vi "ConfigPanel.vi"(8 "ErrorIn":errorcluster, 11 "ClusterIn":T4={"Admin"={"Lvl"=enum."Admin", "Pwd"=""}, "RTConfig"={"Arm"=FALSE, "Number"=0.0, "String"=""}, "SMS"={"Enbl?"=FALSE, "Addr"=[]}, "FPGA"={"Target"=enum."4", "Channel"=enum."4", "Ref1"=refnum, "Ref2"=refnum}, "Config"={"UsrCfg"={"Paths"={"CfgFile"=path "", "LogFolder"=path "", "LogFile"=path "", "NAS path"=path "", "ThreshFile"=path "", "RedunFolder"=path ""}, "SampleRate"=12500.0}, "FP_User"={"#NoiseSums"=1, "Max_df"=1, "AvgAvg"=FALSE, "#Avg"=1, "AutoCenter"=FALSE, "Inclin"={"Vmin"=0.0, "Vmax"=0.0, "Angle_min"=0.0, "Angle_max"=0.0, "Offset"=0.0, "Pos_Neg"=FALSE}, "1"={"Cal_"={"Fine"=0.999969482421875, "Coarse_"=10000.0}, "Beac"={"Fine"=4194303.0, "Coarse_"=1.0}, "Scale"={"Step4"=10000.0, "Step5"=4194303.0, "Step6"=1.0, "Step7"=10000.0}, "Offset"=1.0, "Scale_Noise"=12500.0, "Scale_Step1"=65535.0, "Scale_In_RT"=1.0, "ScaleMeas"=0.999969482421875, "FreqsToRemove"=[0, 1633], "Width"=[0, 1633], "ScaleMeasEnum"=enum."50", "FilterEnab"=enum."Step 1"}, "2"={"Cal_"={"Fine"=0.000213623046875, "Coarse_"=4194303.0}, "Beac"={"Fine"=0.000213623046875, "Coarse_"=4194303.0}, "Scale"={"Step4"=0.0, "Step5"=4194303.0, "Step6"=1.0, "Step7"=10000.0}, "Offset"=0.0, "Scale_Noise"=4194303.0, "Scale_Step1"=65535.0, "Scale_In_RT"=1.0, "ScaleMeas"=0.999969482421875, "FreqsToRemove"=[0, 1633], "Width"=[0, 1633], "ScaleMeasEnum"=enum."50", "FilterEnab"=enum."Step 1"}, "3"={"Cal_"={"Fine"=0.000213623046875, "Coarse_"=4194303.0}, "Beac"={"Fine"=0.000213623046875, "Coarse_"=4194303.0}, "Scale"={"Step4"=0.0, "Step5"=4194303.0, "Step6"=1.0, "Step7"=10000.0}, "Offset"=0.0, "Scale_Noise"=4194303.0, "Scale_Step1"=65535.0, "Scale_In_RT"=1.0, "ScaleMeas"=0.999969482421875, "FreqsToRemove"=[0, 1633], "Width"=[0, 1633], "ScaleMeasEnum"=enum."50", "FilterEnab"=enum."Step 1"}, "4"={"Cal_"={"Fine"=0.000213623046875, "Coarse_"=4194303.0}, "Beac"={"Fine"=0.000213623046875, "Coarse_"=4194303.0}, "Scale"={"Step4"=0.0, "Step5"=4194303.0, "Step6"=1.0, "Step7"=10000.0}, "Offset"=0.0, "Scale_Noise"=4194303.0, "Scale_Step1"=1.0, "Scale_In_RT"=10000.0, "ScaleMeas"=0.999969482421875, "FreqsToRemove"=[0, 1633], "Width"=[0, 1633], "ScaleMeasEnum"=enum."50", "FilterEnab"=enum."Step 1"}, "Target to Probe"=enum."4", "SNR_Thresh"=1.0, "Paths"={"CfgFile"=path "", "LogFolder"=path "", "LogFile"=path "", "NAS path"=path "", "ThreshFile"=path "", "RedunFolder"=path ""}, "Connex_Location"="", "SimulateFPGA"=FALSE, "Deadband"=0.0}}, "Stat"={"SysState"=enum."Init", "TrackRate"=FALSE, "AutoCentr"=FALSE}, "Alarm"={"TC13"={"Enbl"=FALSE, "ErrsAndWarns"={0.0, 5.663716814159292, 7.168141592920354, 8.584070796460177}}, "AI1"={"Enbl"=FALSE, "ErrsAndWarns"={0.0, 5.663716814159292, 7.168141592920354, 8.584070796460177}}, "AI2"={"Enbl"=FALSE, "ErrsAndWarns"={0.0, 5.663716814159292, 7.168141592920354, 8.584070796460177}}, "AI3"={"Enbl"=FALSE, "ErrsAndWarns"={0.0, 5.663716814159292, 7.168141592920354, 8.584070796460177}}, "AI4"={"Enbl"=FALSE, "ErrsAndWarns"={0.0, 5.663716814159292, 7.168141592920354, 8.584070796460177}}, "AI5"={"Enbl"=FALSE, "ErrsAndWarns"={0.0, 5.663716814159292, 7.168141592920354, 8.584070796460177}}, "AI6"={"Enbl"=FALSE, "ErrsAndWarns"={0.0, 5.663716814159292, 7.168141592920354, 8.584070796460177}}, "AI18"={"Enbl"=FALSE, "ErrsAndWarns"={0.0, 5.663716814159292, 7.168141592920354, 8.584070796460177}}, "AI19"={"Enbl"=FALSE, "ErrsAndWarns"={0.0, 5.663716814159292, 7.168141592920354, 8.584070796460177}}, "TE1"={"Enbl"=FALSE, "ErrsAndWarns"={0.0, 5.663716814159292, 7.168141592920354, 8.584070796460177}}, "TE2"={"Enbl"=TRUE, "ErrsAndWarns"={0.0, 5.663716814159292, 7.168141592920354, 8.584070796460177}}, "TE3"={"Enbl"=FALSE, "ErrsAndWarns"={0.0, 5.663716814159292, 7.168141592920354, 8.584070796460177}}, "ADAM1"={"Enbl"=FALSE, "ErrsAndWarns"={0.0, 5.663716814159292, 7.168141592920354, 8.584070796460177}}, "ADAM2"={"Enbl"=FALSE, "ErrsAndWarns"={0.0, 5.663716814159292, 7.168141592920354, 8.584070796460177}}, "ADAM3"={"Enbl"=FALSE, "ErrsAndWarns"={0.0, 5.663716814159292, 7.168141592920354, 8.584070796460177}}, "ADAM4"={"Enbl"=FALSE, "ErrsAndWarns"={0.0, 5.663716814159292, 7.168141592920354, 8.584070796460177}}, "72CoBeacFreq"={"Enbl"=FALSE, "ErrsAndWarns"={0.0, 5.663716814159292, 7.168141592920354, 8.584070796460177}}, "72CoCalFreq"={"Enbl"=FALSE, "ErrsAndWarns"={0.0, 5.663716814159292, 7.168141592920354, 8.584070796460177}}, "84CoBeacFreq"={"Enbl"=FALSE, "ErrsAndWarns"={0.0, 5.663716814159292, 7.168141592920354, 8.584070796460177}}, "84CoCalFreq"={"Enbl"=FALSE, "ErrsAndWarns"={0.0, 5.663716814159292, 7.168141592920354, 8.584070796460177}}, "72Co_CalTonePwr"={"Enbl"=FALSE, "ErrsAndWarns"={0.0, 5.663716814159292, 7.168141592920354, 8.584070796460177}}, "72X_CalTonePwr"={"Enbl"=FALSE, "ErrsAndWarns"={0.0, 5.663716814159292, 7.168141592920354, 8.584070796460177}}, "84Co_CalTonePwr"={"Enbl"=FALSE, "ErrsAndWarns"={0.0, 5.663716814159292, 7.168141592920354, 8.584070796460177}}, "84X_CalTonePwr"={"Enbl"=FALSE, "ErrsAndWarns"={0.0, 5.663716814159292, 7.168141592920354, 8.584070796460177}}}} {"Alarm"."84X_CalTonePwr"."ErrsAndWarns" scale=-120.0..-45.0; "Alarm"."72X_CalTonePwr"."ErrsAndWarns" scale=-120.0..-45.0; "Alarm"."84Co_CalTonePwr"."ErrsAndWarns" scale=-120.0..-45.0; "Alarm"."72Co_CalTonePwr"."ErrsAndWarns" scale=-120.0..-45.0; "Alarm"."84CoCalFreq"."ErrsAndWarns" scale=24.9..25.1; "Alarm"."84CoBeacFreq"."ErrsAndWarns" scale=25.5..27.0; "Alarm"."72CoCalFreq"."ErrsAndWarns" scale=24.9..25.1; "Alarm"."72CoBeacFreq"."ErrsAndWarns" scale=25.5..27.0; "Alarm"."ADAM4"."ErrsAndWarns" scale=30.0..52.0; "Alarm"."ADAM3"."ErrsAndWarns" scale=30.0..52.0; "Alarm"."ADAM2"."ErrsAndWarns" scale=30.0..52.0; "Alarm"."ADAM1"."ErrsAndWarns" scale=30.0..52.0; "Alarm"."TE3"."ErrsAndWarns" scale=30.0..52.0; "Alarm"."TE2"."ErrsAndWarns" scale=30.0..52.0; "Alarm"."TE1"."ErrsAndWarns" scale=20.0..52.0; "Alarm"."AI19"."ErrsAndWarns" scale=0.0..60.0; "Alarm"."AI18"."ErrsAndWarns" scale=-10.0..10.0; "Alarm"."AI6"."ErrsAndWarns" scale=0.0..35.0; "Alarm"."AI5"."ErrsAndWarns" scale=0.0..20.0; "Alarm"."AI4"."ErrsAndWarns" scale=0.0..15.0; "Alarm"."AI3"."ErrsAndWarns" scale=0.0..10.0; "Alarm"."AI2"."ErrsAndWarns" scale=0.0..10.0; "Alarm"."TC13"."ErrsAndWarns" scale=-10.0..40.0; "Config"."FP_User"."Deadband" format="%#.0f"}) -> (0 "ErrorOut":errorcluster, 3 "ClusterOut":T4={"Admin"={"Lvl"=enum."Admin", "Pwd"=""}, "RTConfig"={"Arm"=FALSE, "Number"=0.0, "String"=""}, "SMS"={"Enbl?"=FALSE, "Addr"=[]}, "FPGA"={"Target"=enum."4", "Channel"=enum."4", "Ref1"=refnum, "Ref2"=refnum}, "Config"={"UsrCfg"={"Paths"={"CfgFile"=path "", "LogFolder"=path "", "LogFile"=path "", "NAS path"=path "", "ThreshFile"=path "", "RedunFolder"=path ""}, "SampleRate"=12500.0}, "FP_User"={"#NoiseSums"=1, "Max_df"=1, "AvgAvg"=FALSE, "#Avg"=1, "AutoCenter"=FALSE, "Inclin"={"Vmin"=0.0, "Vmax"=0.0, "Angle_min"=0.0, "Angle_max"=0.0, "Offset"=0.0, "Pos_Neg"=FALSE}, "1"={"Cal_"={"Fine"=0.999969482421875, "Coarse_"=10000.0}, "Beac"={"Fine"=4194303.0, "Coarse_"=1.0}, "Scale"={"Step4"=10000.0, "Step5"=4194303.0, "Step6"=1.0, "Step7"=10000.0}, "Offset"=1.0, "Scale_Noise"=12500.0, "Scale_Step1"=65535.0, "Scale_In_RT"=1.0, "ScaleMeas"=0.999969482421875, "FreqsToRemove"=[0, 1633], "Width"=[0, 1633], "ScaleMeasEnum"=enum."50", "FilterEnab"=enum."Step 1"}, "2"={"Cal_"={"Fine"=0.000213623046875, "Coarse_"=4194303.0}, "Beac"={"Fine"=0.000213623046875, "Coarse_"=4194303.0}, "Scale"={"Step4"=0.0, "Step5"=4194303.0, "Step6"=1.0, "Step7"=10000.0}, "Offset"=0.0, "Scale_Noise"=4194303.0, "Scale_Step1"=65535.0, "Scale_In_RT"=1.0, "ScaleMeas"=0.999969482421875, "FreqsToRemove"=[0, 1633], "Width"=[0, 1633], "ScaleMeasEnum"=enum."50", "FilterEnab"=enum."Step 1"}, "3"={"Cal_"={"Fine"=0.000213623046875, "Coarse_"=4194303.0}, "Beac"={"Fine"=0.000213623046875, "Coarse_"=4194303.0}, "Scale"={"Step4"=0.0, "Step5"=4194303.0, "Step6"=1.0, "Step7"=10000.0}, "Offset"=0.0, "Scale_Noise"=4194303.0, "Scale_Step1"=65535.0, "Scale_In_RT"=1.0, "ScaleMeas"=0.999969482421875, "FreqsToRemove"=[0, 1633], "Width"=[0, 1633], "ScaleMeasEnum"=enum."50", "FilterEnab"=enum."Step 1"}, "4"={"Cal_"={"Fine"=0.000213623046875, "Coarse_"=4194303.0}, "Beac"={"Fine"=0.000213623046875, "Coarse_"=4194303.0}, "Scale"={"Step4"=0.0, "Step5"=4194303.0, "Step6"=1.0, "Step7"=10000.0}, "Offset"=0.0, "Scale_Noise"=4194303.0, "Scale_Step1"=1.0, "Scale_In_RT"=10000.0, "ScaleMeas"=0.999969482421875, "FreqsToRemove"=[0, 1633], "Width"=[0, 1633], "ScaleMeasEnum"=enum."50", "FilterEnab"=enum."Step 1"}, "Target to Probe"=enum."4", "SNR_Thresh"=1.0, "Paths"={"CfgFile"=path "", "LogFolder"=path "", "LogFile"=path "", "NAS path"=path "", "ThreshFile"=path "", "RedunFolder"=path ""}, "Connex_Location"="", "SimulateFPGA"=FALSE, "Deadband"=0.0}}, "Stat"={"SysState"=enum."Init", "TrackRate"=FALSE, "AutoCentr"=FALSE}, "Alarm"={"TC13"={"Enbl"=FALSE, "ErrsAndWarns"={0.0, 5.663716814159292, 7.168141592920354, 8.584070796460177}}, "AI1"={"Enbl"=FALSE, "ErrsAndWarns"={0.0, 5.663716814159292, 7.168141592920354, 8.584070796460177}}, "AI2"={"Enbl"=FALSE, "ErrsAndWarns"={0.0, 5.663716814159292, 7.168141592920354, 8.584070796460177}}, "AI3"={"Enbl"=FALSE, "ErrsAndWarns"={0.0, 5.663716814159292, 7.168141592920354, 8.584070796460177}}, "AI4"={"Enbl"=FALSE, "ErrsAndWarns"={0.0, 5.663716814159292, 7.168141592920354, 8.584070796460177}}, "AI5"={"Enbl"=FALSE, "ErrsAndWarns"={0.0, 5.663716814159292, 7.168141592920354, 8.584070796460177}}, "AI6"={"Enbl"=FALSE, "ErrsAndWarns"={0.0, 5.663716814159292, 7.168141592920354, 8.584070796460177}}, "AI18"={"Enbl"=FALSE, "ErrsAndWarns"={0.0, 5.663716814159292, 7.168141592920354, 8.584070796460177}}, "AI19"={"Enbl"=FALSE, "ErrsAndWarns"={0.0, 5.663716814159292, 7.168141592920354, 8.584070796460177}}, "TE1"={"Enbl"=FALSE, "ErrsAndWarns"={0.0, 5.663716814159292, 7.168141592920354, 8.584070796460177}}, "TE2"={"Enbl"=TRUE, "ErrsAndWarns"={0.0, 5.663716814159292, 7.168141592920354, 8.584070796460177}}, "TE3"={"Enbl"=FALSE, "ErrsAndWarns"={0.0, 5.663716814159292, 7.168141592920354, 8.584070796460177}}, "ADAM1"={"Enbl"=FALSE, "ErrsAndWarns"={0.0, 5.663716814159292, 7.168141592920354, 8.584070796460177}}, "ADAM2"={"Enbl"=FALSE, "ErrsAndWarns"={0.0, 5.663716814159292, 7.168141592920354, 8.584070796460177}}, "ADAM3"={"Enbl"=FALSE, "ErrsAndWarns"={0.0, 5.663716814159292, 7.168141592920354, 8.584070796460177}}, "ADAM4"={"Enbl"=FALSE, "ErrsAndWarns"={0.0, 5.663716814159292, 7.168141592920354, 8.584070796460177}}, "72CoBeacFreq"={"Enbl"=FALSE, "ErrsAndWarns"={0.0, 5.663716814159292, 7.168141592920354, 8.584070796460177}}, "72CoCalFreq"={"Enbl"=FALSE, "ErrsAndWarns"={0.0, 5.663716814159292, 7.168141592920354, 8.584070796460177}}, "84CoBeacFreq"={"Enbl"=FALSE, "ErrsAndWarns"={0.0, 5.663716814159292, 7.168141592920354, 8.584070796460177}}, "84CoCalFreq"={"Enbl"=FALSE, "ErrsAndWarns"={0.0, 5.663716814159292, 7.168141592920354, 8.584070796460177}}, "72Co_CalTonePwr"={"Enbl"=FALSE, "ErrsAndWarns"={0.0, 5.663716814159292, 7.168141592920354, 8.584070796460177}}, "72X_CalTonePwr"={"Enbl"=FALSE, "ErrsAndWarns"={0.0, 5.663716814159292, 7.168141592920354, 8.584070796460177}}, "84Co_CalTonePwr"={"Enbl"=FALSE, "ErrsAndWarns"={0.0, 5.663716814159292, 7.168141592920354, 8.584070796460177}}, "84X_CalTonePwr"={"Enbl"=FALSE, "ErrsAndWarns"={0.0, 5.663716814159292, 7.168141592920354, 8.584070796460177}}}} {"Alarm"."84X_CalTonePwr"."ErrsAndWarns" scale=-120.0..-45.0; "Alarm"."72X_CalTonePwr"."ErrsAndWarns" scale=-120.0..-45.0; "Alarm"."84Co_CalTonePwr"."ErrsAndWarns" scale=-120.0..-45.0; "Alarm"."72Co_CalTonePwr"."ErrsAndWarns" scale=-120.0..-45.0; "Alarm"."84CoCalFreq"."ErrsAndWarns" scale=24.9..25.1; "Alarm"."84CoBeacFreq"."ErrsAndWarns" scale=25.5..27.0; "Alarm"."72CoCalFreq"."ErrsAndWarns" scale=24.9..25.1; "Alarm"."72CoBeacFreq"."ErrsAndWarns" scale=25.5..27.0; "Alarm"."ADAM4"."ErrsAndWarns" scale=30.0..52.0; "Alarm"."ADAM3"."ErrsAndWarns" scale=30.0..52.0; "Alarm"."ADAM2"."ErrsAndWarns" scale=30.0..52.0; "Alarm"."ADAM1"."ErrsAndWarns" scale=30.0..52.0; "Alarm"."TE3"."ErrsAndWarns" scale=30.0..52.0; "Alarm"."TE2"."ErrsAndWarns" scale=30.0..52.0; "Alarm"."TE1"."ErrsAndWarns" scale=20.0..52.0; "Alarm"."AI19"."ErrsAndWarns" scale=0.0..60.0; "Alarm"."AI18"."ErrsAndWarns" scale=-10.0..10.0; "Alarm"."AI6"."ErrsAndWarns" scale=0.0..35.0; "Alarm"."AI5"."ErrsAndWarns" scale=0.0..20.0; "Alarm"."AI4"."ErrsAndWarns" scale=0.0..15.0; "Alarm"."AI3"."ErrsAndWarns" scale=0.0..10.0; "Alarm"."AI2"."ErrsAndWarns" scale=0.0..10.0; "Alarm"."TC13"."ErrsAndWarns" scale=-10.0..40.0; "Config"."FP_User"."Deadband" format="%#.0f"})   [LabVIEW 2018]
doc: "This modal dialog allows the user to enter configuration data that is saved from one run to the next. This is useful for maintaining information such as instrument settings, display preferences, etc.\n\nIn general, each control on this panel should be Type-Def'd and saved to an INI file whenever the user clicks the OK button.\n\nCopyright © 2019 Epimedia, Inc. All Rights Reserved.\n\nThe Epimedia Application Library is Copyright © 2009-2019 Epimedia, Inc. \nAll Rights Reserved. Used under license."
uses:
  Controls/MasterCluster.ctl
  Controls/Clusts/AdminCluster.ctl
  Controls/UserLevelEnum.ctl
  Controls/RT_Config.ctl
  Controls/SMSDataCluster.ctl
  Controls/Clusts/FPGA_Config_Clust.ctl
  Controls/Enums/TargetNumber.ctl
  Controls/Clusts/Config_Clust.ctl
  Controls/Clusts/UserConfig.ctl
  Controls/PathsCluster.ctl
  Controls/Clusts/FrontPanel_UserConfig.ctl
  Controls/Clusts/Inclinometer_User_Cfg.ctl
  Controls/Clusts/FP_UserTargetConfig.ctl
  Controls/Clusts/FreqShift.ctl
  Controls/Clusts/FPGA_Scale.ctl
  Controls/Enums/ScaleMeasure.ctl
  Controls/RadioButtons/FilterEnableRadio.ctl
  Controls/SystemStatusCluster.ctl
  Controls/SystemStateEnum.ctl
  Controls/Clusts/AlarmSettingsClust.ctl
  Controls/Clusts/AlarmThresh_OneChan.ctl
  Queue/ConfigQueueElements.ctl
panel:
  in  "Paths":T1
  in  "User":T2
  in  "Cancel":bool
  in  "OK":bool
  # "Copyright © 2019 Epimedia, Inc. All Rights Reserved.\n\nThe Epimedia Application Library is Copyright © 2009-2019 Epimedia, Inc. \nAll Rights Reserved. Used under license."
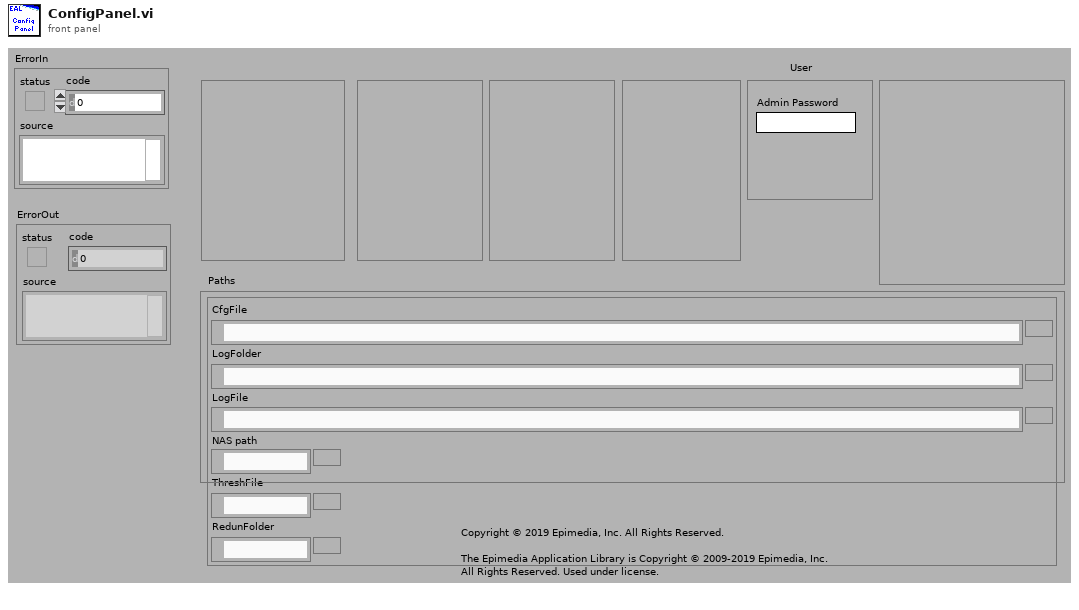
[diagram p1: front panel]
types:
  T1 = typedef "PathsCluster.ctl" = cluster{"CfgFile":path, "LogFolder":path, "LogFile":path, "NAS path":path, "ThreshFile":path, "RedunFolder":path}
  T2 = typedef "AdminCluster.ctl" = cluster{"Lvl":T3, "Pwd":string}
  T3 = typedef "UserLevelEnum.ctl" = enum16{"Admin", "Operator"}
  T4 = typedef "MasterCluster.ctl" = cluster{"Admin":T2, "RTConfig":T5, "SMS":T6, "FPGA":T7, "Config":T9, "Stat":T18, "Alarm":T20}
  T5 = typedef "RT_Config.ctl" = cluster{"Arm":bool, "Number":dbl, "String":string}
  T6 = typedef "SMSDataCluster.ctl" = cluster{"Enbl?":bool, "Addr":string[]}
  T7 = typedef "FPGA_Config_Clust.ctl" = cluster{"Target":T8, "Channel":T8, "Ref1":refnum<k20>, "Ref2":refnum<k20>}
  T8 = typedef "TargetNumber.ctl" = enum16{"1", "2", "3", "4"}
  T9 = typedef "Config_Clust.ctl" = cluster{"UsrCfg":T10, "FP_User":T11}
  T10 = typedef "UserConfig.ctl" = cluster{"Paths":T1, "SampleRate":dbl}
  T11 = typedef "FrontPanel_UserConfig.ctl" = cluster{"#NoiseSums":u32, "Max_df":u32, "AvgAvg":bool, "#Avg":u16, "AutoCenter":bool, "Inclin":T12, "1":T13, "2":T13, "3":T13, "4":T13, "Target to Probe":T8, "SNR_Thresh":dbl, "Paths":T1, "Connex_Location":string, "SimulateFPGA":bool, "Deadband":dbl}
  T12 = typedef "Inclinometer_User_Cfg.ctl" = cluster{"Vmin":dbl, "Vmax":dbl, "Angle_min":dbl, "Angle_max":dbl, "Offset":dbl, "Pos_Neg":bool}
  T13 = typedef "FP_UserTargetConfig.ctl" = cluster{"Cal_":T14, "Beac":T14, "Scale":T15, "Offset":fxp<+/-,16,16>, "Scale_Noise":fxp<+/-,30,30>, "Scale_Step1":fxp<+/-,17,17>, "Scale_In_RT":ext, "ScaleMeas":fxp<+/-,16,1>, "FreqsToRemove":i32[], "Width":i32[], "ScaleMeasEnum":T16, "FilterEnab":T17}
  T14 = typedef "FreqShift.ctl" = cluster{"Fine":dbl, "Coarse_":dbl}
  T15 = typedef "FPGA_Scale.ctl" = cluster{"Step4":fxp<+/-,23,23>, "Step5":fxp<+/-,23,23>, "Step6":fxp<+/-,23,23>, "Step7":fxp<+/-,23,23>}
  T16 = typedef "ScaleMeasure.ctl" = enum16{"1", "10", "50", "42"}
  T17 = typedef "FilterEnableRadio.ctl" = enum32{"None", "Step 1", "Frequency Shift", "Step 4", "Step 5", "Step 6", "Step 7"}
  T18 = typedef "SystemStatusCluster.ctl" = cluster{"SysState":T19, "TrackRate":bool, "AutoCentr":bool}
  T19 = typedef "SystemStateEnum.ctl" = enum16{"Init", "Idle", "Running", "System Fault", "System Error", "Exit"}
  T20 = typedef "AlarmSettingsClust.ctl" = cluster{"TC13":T21, "AI1":T21, "AI2":T21, "AI3":T21, "AI4":T21, "AI5":T21, "AI6":T21, "AI18":T21, "AI19":T21, "TE1":T21, "TE2":T21, "TE3":T21, "ADAM1":T21, "ADAM2":T21, "ADAM3":T21, "ADAM4":T21, "72CoBeacFreq":T21, "72CoCalFreq":T21, "84CoBeacFreq":T21, "84CoCalFreq":T21, "72Co_CalTonePwr":T21, "72X_CalTonePwr":T21, "84Co_CalTonePwr":T21, "84X_CalTonePwr":T21}
  T21 = typedef "AlarmThresh_OneChan.ctl" = cluster{"Enbl":bool, "ErrsAndWarns":cluster{dbl, dbl, dbl, dbl}}
  T22 = typedef "ConfigQueueElements.ctl" = enum16{"Initialize", "OK", "Cancel"}
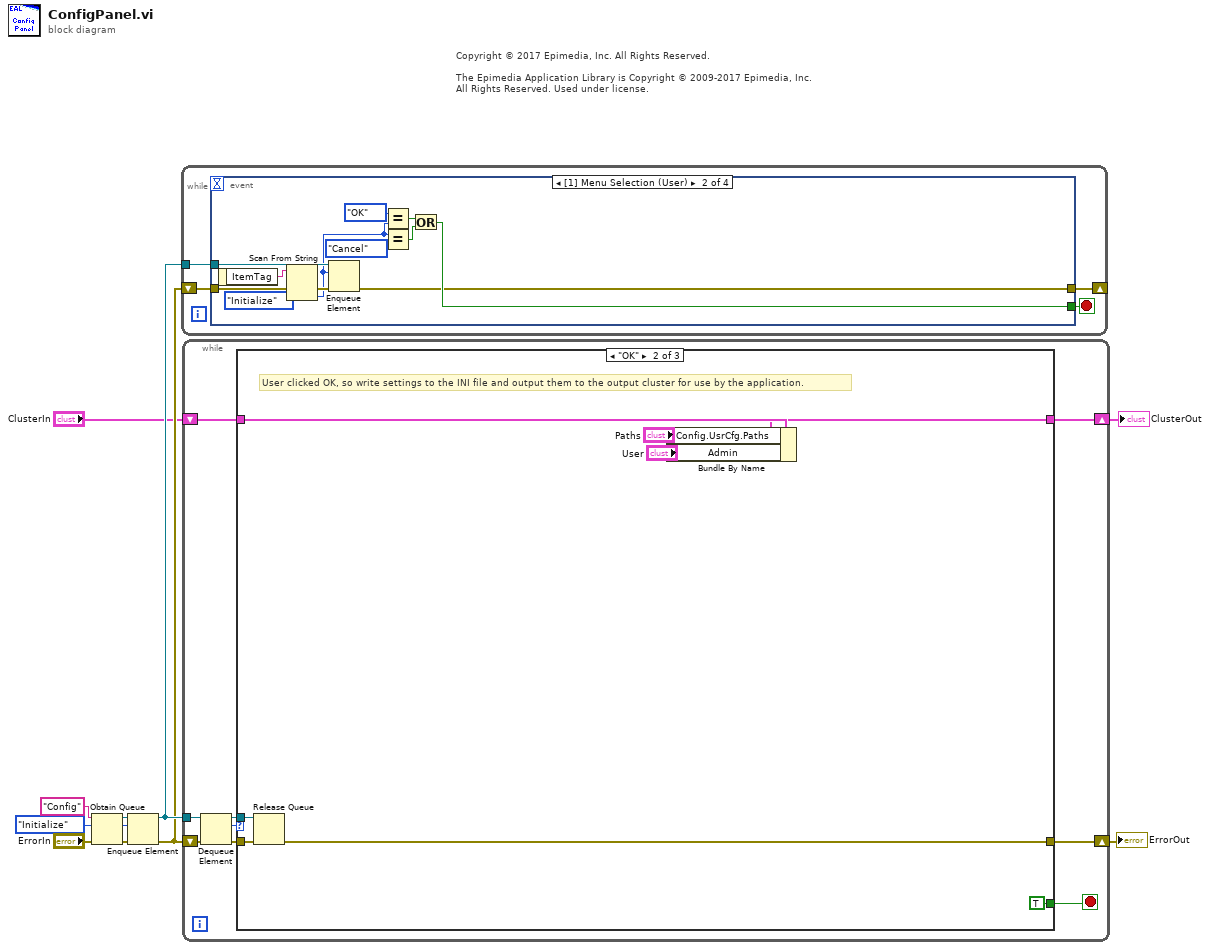
[diagram p0: block diagram]
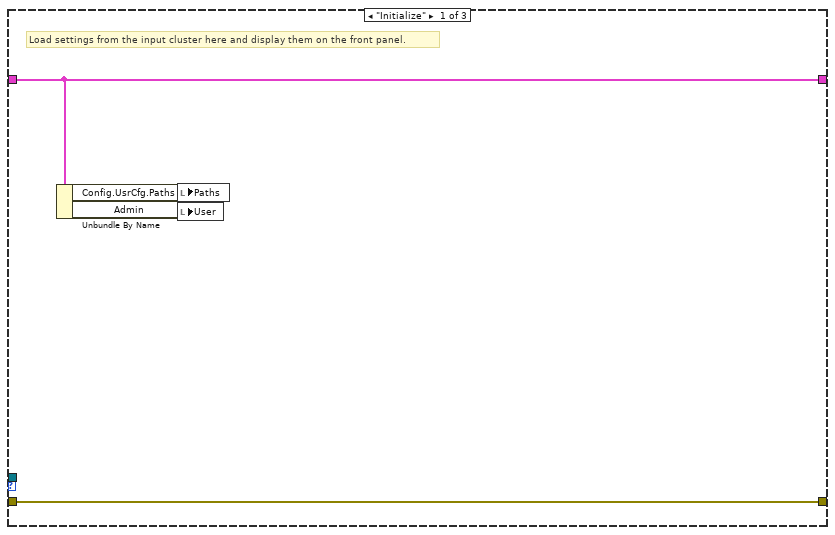
[diagram p2: hidden frame]
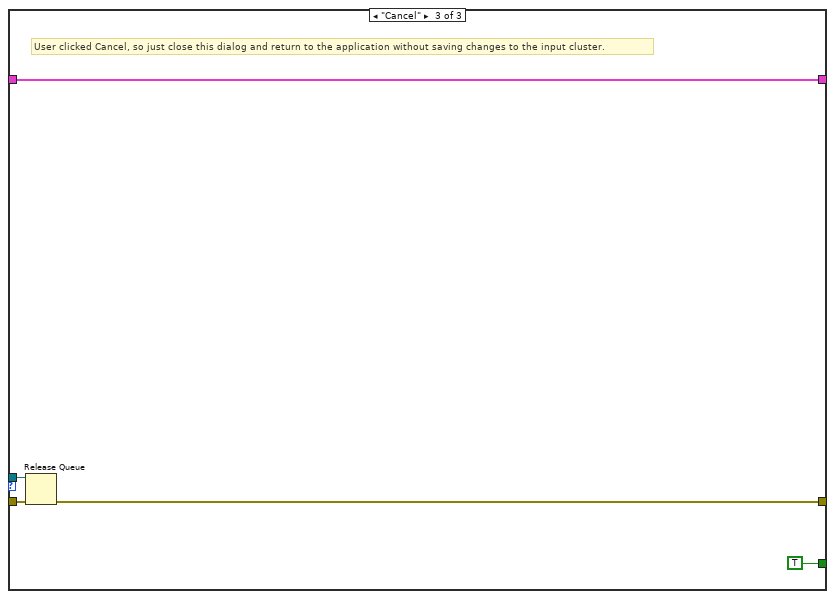
[diagram p3: hidden frame]
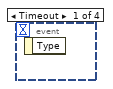
[diagram p4: hidden frame]
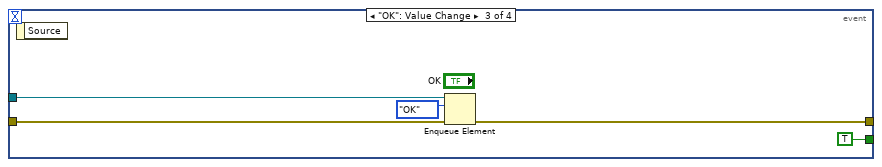
[diagram p5: hidden frame]
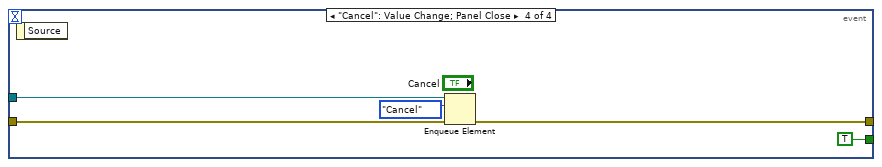
[diagram p6: hidden frame]
diagram:
  w1 = ConfigQueueElements."Initialize" ("MainQueueElements")
  # "Copyright © 2017 Epimedia, Inc. All Rights Reserved.\n\nThe Epimedia Application Library is Copyright © 2009-2017 Epimedia, Inc. \nAll Rights Reserved. Used under license."
  n1 = Obtain Queue(name (unnamed)="Config", element data type=w1, error in (no error)="ErrorIn") -> (queue out=w7:refnum<queue>, error out=w8:errorcluster)  [unwired: 2 in, 1 out]
  n2 = Enqueue Element(queue=w7, element=w1, error in (no error)=w8) -> (queue out=w6:refnum<queue>, error out=w5:errorcluster)  [unwired: 2 out]
  n3 = while {
    tunnel: w6 -> [w13]
    shift-right: [w12] -> _
    shift-left: w5 -> [w14]
    stop <- w11 stop-if-true
    n4 = event shown="[1] Menu Selection (User)" {
      selector: _ -> [_ _ _ _]
      dyn-events: _ -> [_ _ _ _]
      timeout: _ -> [_ _ _ _]
      tunnel: w14 -> [_ w22 w31 w36]
      tunnel: w13 -> [_ w21 w30 w35]
      tunnel: [_ w16 w29 w34] -> w12
      tunnel: [_ w18 TRUE TRUE] -> w11
      event Timeout {
        n5 = event-data() -> ()  [unwired: 2 out]
      }
      event Menu Selection (User) {
        n6 = event-data() -> ("ItemTag"=w23:string)  [unwired: 1 out]
        n7 = Scan From String(input string=w23, error in=w22, default 1=ConfigQueueElements."Initialize" ("MainQueueElements")) -> (error out=w26:errorcluster, output 1=w15:T22)  [unwired: 2 in, 2 out]
        n8 = Enqueue Element(queue=w21, element=w15, error in (no error)=w26) -> (error out=w16:errorcluster)  [unwired: 3 out]
        n9 = Equal?(x=ConfigQueueElements."OK" ("MainQueueElements"), y=w15) -> (x = y?=w20:bool)
        n10 = Equal?(x=w15, y=ConfigQueueElements."Cancel" ("MainQueueElements")) -> (x = y?=w19:bool)
        n11 = Or(x=w20, y=w19) -> (x .or. y?=w18:bool)
      }
      event "OK": Value Change {
        n12 = event-data() -> ()  [unwired: 2 out]
        n13 = Enqueue Element(queue=w30, element=ConfigQueueElements."OK", error in (no error)=w31) -> (error out=w29:errorcluster)  [unwired: 3 out]
      }
      event "Cancel": Value Change; Panel Close {
        n14 = event-data() -> ()  [unwired: 2 out]
        n15 = Enqueue Element(queue=w35, element=ConfigQueueElements."Cancel", error in (no error)=w36) -> (error out=w34:errorcluster)  [unwired: 3 out]
      }
    }
  }
  n16 = while {
    shift-right: [w37] -> w3
    shift-left: w5 -> [w45]
    tunnel: w6 -> [w44]
    shift-right: [w39] -> w4
    shift-left: "ClusterIn" -> [w40]
    stop <- w38 stop-if-true
    n17 = Dequeue Element(queue=w44, error in (no error)=w45) -> (queue out=w42:refnum<queue>, element=w41:T22, error out=w43:errorcluster)  [unwired: 2 out]
    n18 = case shown="\"OK\"" w41 {
      tunnel: w43 -> [w46 w57 w62]
      tunnel: w42 -> [_ w56 w61]
      tunnel: [w46 w50 w60] -> w37
      tunnel: [w49 w53 w58] -> w39
      tunnel: w40 -> [w49 w54 w58]
      tunnel: [_ TRUE TRUE] -> w38
      frame "Initialize" {
        # "Load settings from the input cluster here and display them on the front panel."
        n19 = Unbundle By Name(w49) -> ("Config.UsrCfg.Paths"=w47:T1, "Admin"=w48:T2)
        n20 = local write "Paths"(w47) -> ()
        n21 = local write "User"(w48) -> ()
      }
      frame "OK" {
        # "User clicked OK, so write settings to the INI file and output them to the output cluster for use by the application."
        n22 = Release Queue(queue=w56, error in (no error)=w57) -> (error out=w50:errorcluster)  [unwired: 3 out]
        n23 = Bundle By Name(cluster=w54, "Config.UsrCfg.Paths"="Paths", "Admin"="User") -> (w53:T4)
      }
      frame "Cancel" {
        # "User clicked Cancel, so just close this dialog and return to the application without saving changes to the input cluster."
        n24 = Release Queue(queue=w61, error in (no error)=w62) -> (error out=w60:errorcluster)  [unwired: 3 out]
      }
    }
  }
  "ErrorOut" <- w3
  "ClusterOut" <- w4
